vi "Add Attribute Integer.vi"(8 "data":i32[](array[numeric]), 9 "Attribute name":string, 10 "loc_id":i32, 11 "error in (no error)":errorcluster) -> (3 "error out":errorcluster)   [LabVIEW 2014, in "HDF5Tools.lvlib"]
uses:
  HDF5Tools.lvlib
  Cajal/private/HDF5Tools32/Release/hdf5_hl.dll
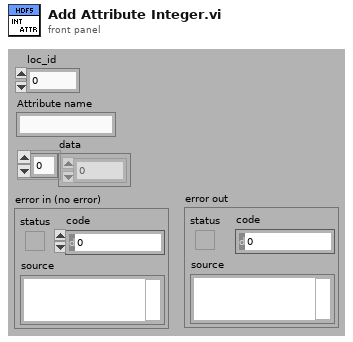
[diagram p1: front panel]
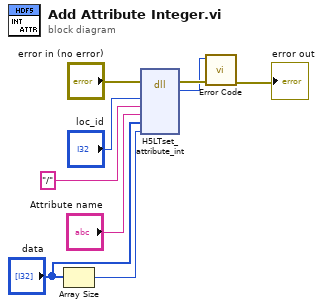
[diagram p0: block diagram]
diagram:
  n1 = Array Size(array="data") -> (size(s)=w4:i32)
  n2 = dll-call lib="Z:/users/Manolis/Labview/Cajal/private/HDF5Tools32/Release/hdf5_hl.dll" fn="H5LTset_attribute_int"(error in="error in (no error)", "loc_id"="loc_id", "obj_name"="/", "attr_name"="Attribute name", "data"="data", "size"=w4) -> (error out=w3:errorcluster, "error"=w1:i32)  [unwired: 7 in, 1 out]
  n3 = call "Error Code.vi"("Error in"=w3, "Error code"=w1) -> ("Error out"=→"error out":errorcluster)  [unwired: 9 in]
